vi "WIDTH.vi"() -> (0 "WIDTH":i16=400)   [LabVIEW 2020]
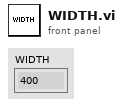
[diagram p1: front panel]
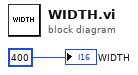
[diagram p0: block diagram]
diagram:
  "WIDTH" <- i16 400
